vi "Write DO_index.vi"(6 "Find all":bool=TRUE, 9 "Heater":string, 10 "EnumsDO":string[](array[string]), 11 "Heater in":refnum<class "Heater.lvclass">) -> (2 "Find":bool, 3 "Heater out":refnum<class "Heater.lvclass">)   [LabVIEW 2019, in "Heating.lvlib" / "Heater.lvclass"]
uses:
  Heater.lvclass
  Heater.lvclass/Heater.ctl
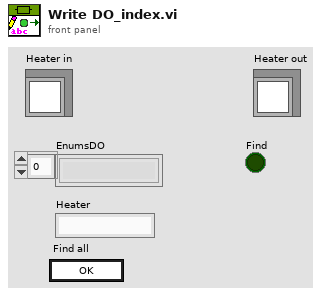
[diagram p1: front panel]
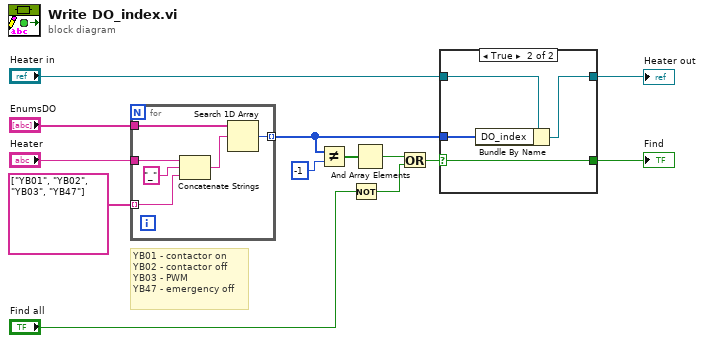
[diagram p0: block diagram]
diagram:
  # "YB01 - contactor on\nYB02 - contactor off\nYB03 - PWM\nYB47 - emergency off"
  n1 = for {
    tunnel: "EnumsDO" -> [w19]
    tunnel: "Heater" -> [w18]
    tunnel: [w16] -> w12 mode=indexing
    tunnel: string[] ["YB01", "YB02", "YB03", "YB47"] -> [w14] mode=indexing
    n2 = Concatenate Strings(w18, "_" ("string"), w14) -> (w17:string)
    n3 = Search 1D Array(1D array=w19, element=w17) -> (index of element=w16:i32)  [unwired: 1 in]
  }
  n4 = Not Equal?(x=w12, y=-1 ("index of element")) -> (x != y?=w9:bool[])
  n5 = Not(x="Find all") -> (.not. x?=w1:bool)
  n6 = And Array Elements(Boolean array=w9) -> (logical AND=w13:bool)
  n7 = Or(x=w13, y=w1) -> (x .or. y?=w3:bool)
  n8 = case shown="True" w3 {
    selector: w3 -> [_ w23]
    tunnel: w12 -> [_ w24]
    tunnel: [_ w23] -> w6
    tunnel: "Heater in" -> [w20 w22]
    tunnel: [w20 w21] -> w7
    frame False {
    }
    frame True {
      n9 = Bundle By Name(cluster=w22, "DO_index"=w24) -> (w21:refnum<class "Heater.lvclass">)
    }
  }
  "Heater out" <- w7
  "Find" <- w6
